vi "Stop Core.vi"(10 "final error code":i32, 11 "SCADA in":refnum<class "SCADA.lvclass">) -> (3 "SCADA out":refnum<class "SCADA.lvclass">)   [LabVIEW 2015, in "SCADA Core.lvlib" / "SCADA.lvclass"]
doc: "(<B>Filename</B>: Actor Framework.lvlib:Actor.lvclass:Stop Core.vi)\n\nDefines what the actor does before it stops. Use the <B>final error code</B> input to determine whether the actor shut down in response to an error.\n\nBy default, this method does nothing. A descendant class may override it to define behavior, such as shutting down any processes the actor initiated in its override of the Actor Core method."
uses:
  SCADA.lvclass
  <vilib>/ActorFramework/Actor/Actor.lvclass
  <vilib>/NI/Tools/Keyed Array/Tools_KeyedArray.lvlib
  <vilib>/ActorFramework/Stop Msg/Stop Msg.lvclass
  Utilities/Status Messaging.llb/Status Messaging.lvlib
  Controls/Queue Selector.ctl
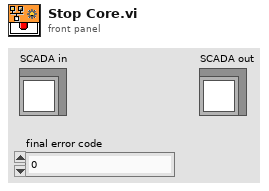
[diagram p1: front panel]
types:
  T1 = typedef "SCADA Core.lvlib/SCADA.lvclass/Queue Selector.ctl" = enum16{"IEDs", "PV", "Generators", "Wind", "Storage", "Relays"}
  T2 = typedef "Tools_KeyedArray.lvlib/KeyedArray.ctl" = cluster{"keys":string[], "values":string[]}
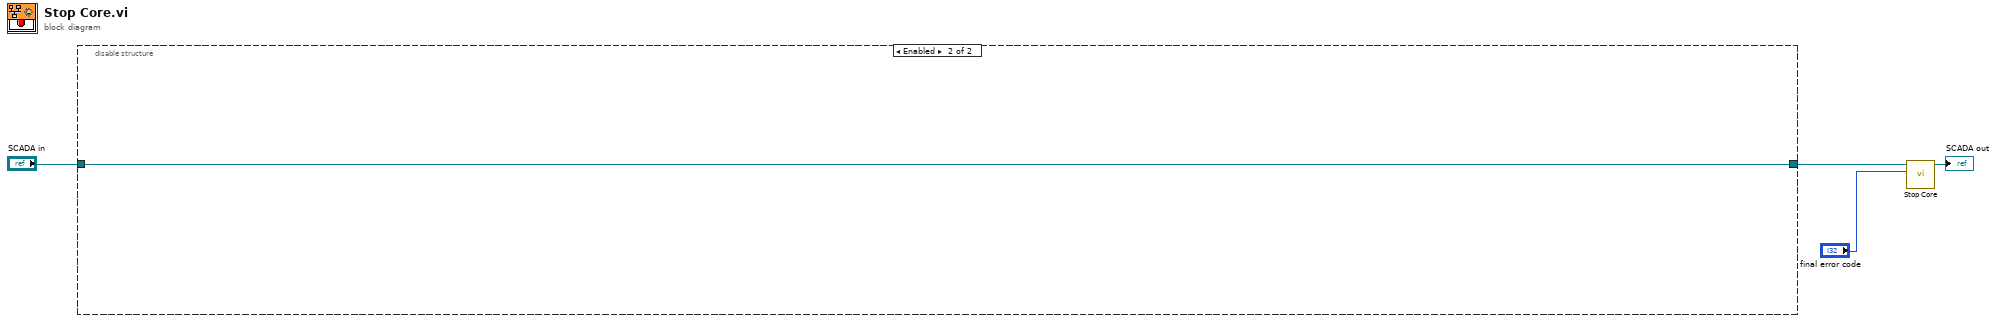
[diagram p0: block diagram]
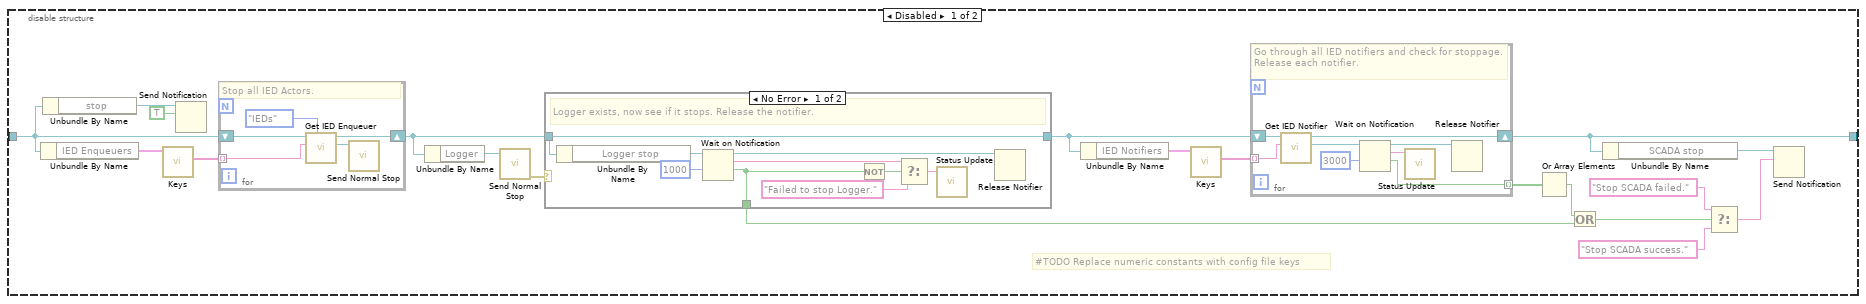
[diagram p2: hidden frame]
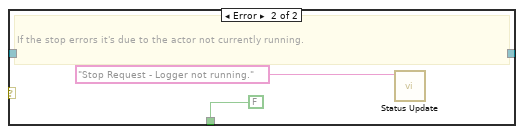
[diagram p3: hidden frame]
diagram:
  n1 = disable-structure shown="Enabled" {
    disable-tunnel: "SCADA in" -> [w20 w50]
    disable-tunnel: [w7 w50] -> w1
    frame Disabled {
      # "#TODO Replace numeric constants with config file keys"
      n2 = Unbundle By Name(w20) -> ("IED Enqueuers"=w22:T2)
      n3 = Unbundle By Name(w20) -> ("stop"=w23:refnum<notifier>)
      n4 = call <vilib>:"Keys.vi"("array in"=w22) -> ("keys"=w21:string[])  [unwired: 5 in, 1 out]
      n5 = Send Notification(notification=TRUE, notifier=w23) -> ()  [unwired: 1 in, 2 out]
      n6 = for {
        tunnel: w21 -> [w48] mode=indexing
        shift-right: [w46] -> w14
        shift-left: w20 -> [w49]
        # "Stop all IED Actors."
        n7 = call "Get IED Enqueuer.vi"("Queue"=Queue_Selector."IEDs", "IED Name"=w48, "SCADA in"=w49) -> ("IED Enqueuer"=w45:refnum<class "Message Enqueuer.lvclass">, "SCADA out"=w46:refnum<class "SCADA.lvclass">)  [unwired: 6 in, 1 out]
        n8 = call <vilib>:"Send Normal Stop.vi"("Message Enqueuer"=w45) -> ()  [unwired: 10 in, 1 out]
      }
      n9 = Unbundle By Name(w14) -> ("Logger"=w16:refnum<class "Message Enqueuer.lvclass">)
      n10 = call <vilib>:"Send Normal Stop.vi"("Message Enqueuer"=w16) -> ("error out"=w15:errorcluster)  [unwired: 10 in]
      n11 = case shown="No Error" w15 {
        tunnel: w14 -> [w33 w36]
        tunnel: [w33 w36] -> w13
        tunnel: [w29 FALSE ("timed out?")] -> w11
        frame No Error {
          # "Logger exists, now see if it stops. Release the notifier."
          n12 = Unbundle By Name(w33) -> ("Logger stop"=w31:refnum<notifier>)
          n13 = Wait on Notification(notifier=w31, timeout in ms (-1)=1000) -> (notifier out=w25:refnum<notifier>, notification=w28:string, timed out?=w29:bool)  [unwired: 2 in, 1 out]
          n14 = Not(x=w29) -> (.not. x?=w30:bool)
          n15 = Select(t=w28, s=w30, f="Failed to stop Logger.") -> (s? t:f=w27:string)
          n16 = call "Status Update.vi"("Status Update"=w27) -> ()  [unwired: 9 in, 2 out]
          n17 = Release Notifier(notifier=w25) -> ()  [unwired: 2 in, 3 out]
        }
        frame Error {
          # "If the stop errors it's due to the actor not currently running."
          n18 = call "Status Update.vi"("Status Update"="Stop Request - Logger not running.") -> ()  [unwired: 9 in, 2 out]
        }
      }
      n19 = Unbundle By Name(w13) -> ("IED Notifiers"=w19:T2)
      n20 = call <vilib>:"Keys.vi"("array in"=w19) -> ("keys"=w18:string[])  [unwired: 5 in, 1 out]
      n21 = for {
        tunnel: w18 -> [w42] mode=indexing
        shift-right: [w43] -> w7
        shift-left: w13 -> [w44]
        tunnel: [w38] -> w17 mode=indexing
        # "Go through all IED notifiers and check for stoppage. Release each notifier."
        n22 = call "Get IED Notifier.vi"("IED Name"=w42, "SCADA in"=w44) -> ("IED Notifier"=w41:refnum<notifier>, "SCADA out"=w43:refnum<class "SCADA.lvclass">)  [unwired: 7 in, 1 out]
        n23 = Wait on Notification(notifier=w41, timeout in ms (-1)=3000) -> (notifier out=w37:refnum<notifier>, notification=w39:string, timed out?=w38:bool)  [unwired: 2 in, 1 out]
        n24 = call "Status Update.vi"("Status Update"=w39) -> ()  [unwired: 9 in, 2 out]
        n25 = Release Notifier(notifier=w37) -> ()  [unwired: 2 in, 3 out]
      }
      n26 = Or Array Elements(Boolean array=w17) -> (logical OR=w12:bool)
      n27 = Or(x=w12, y=w11) -> (x .or. y?=w10:bool)
      n28 = Unbundle By Name(w7) -> ("SCADA stop"=w6:refnum<notifier>)
      n29 = Select(t="Stop SCADA failed." ("notification"), s=w10, f="Stop SCADA success." ("notification")) -> (s? t:f=w5:string)
      n30 = Send Notification(notification=w5, notifier=w6) -> ()  [unwired: 1 in, 2 out]
    }
    frame Enabled {
    }
  }
  n31 = call-parent "Stop Core.vi"("final error code"="final error code", "Actor in"=w1) -> ("Actor out"=→"SCADA out":refnum<class "SCADA.lvclass">)  [unwired: 9 in]
